vi "pH电极校准.vi"() -> ()   [LabVIEW 2016, in "斯坦道多参数.lvlib"]
uses:
  <vilib>/Utility/miscctls.llb/LVPointTypeDef.ctl
  <vilib>/Analysis/NI_AALBase.lvlib
panel:
  out "滤波设定":dbl
  in  "刷新按钮":bool
  out "第三点信号值":dbl
  out "第二点信号值":dbl
  out "第一点信号值":dbl
  out "温度":dbl format="%#.2f"
  out "通讯状态":string
  out "电极状态标志":u16(ring) items=["OK", "第一点校正通过", "第二点校正通过", "校正失败,电极零点超出范围", "校正失败,电极斜率超出范围", "第三点校正通过"]
  in  "三点标液3":u16(ring)=6 caption="标液3" items=["TECH4.00", "TECH7.00", "TECH10.00", "NIST1.68", "NIST4.01", "NIST6.86", "NIST9.18", "NIST12.68"]
  in  "三点标液2":u16(ring)=5 caption="标液2" items=["TECH4.00", "TECH7.00", "TECH10.00", "NIST1.68", "NIST4.01", "NIST6.86", "NIST9.18", "NIST12.68"]
  in  "三点标液1":u16(ring)=4 caption="标液1" items=["TECH4.00", "TECH7.00", "TECH10.00", "NIST1.68", "NIST4.01", "NIST6.86", "NIST9.18", "NIST12.68"]
  out "第三点校准值":dbl
  in  "校准停止":bool
  in  "校准启动":bool
  out "第二点校准值":dbl
  out "第一点校准值":dbl
  out "提示":string
  in  "校准模式":u16(ring) items=["两点校准", "单点校准", "三点校准"]
  out "最小值":sgl format="%#.2f"
  out "最大值":sgl format="%#.2f"
  out "变异系数":dbl format="%#.6f"
  out "standard deviation":dbl caption="标准差" format="%#.2f"
  out "mean":dbl caption="均值" format="%#.2f"
  out "波形图表":sgl(graph) caption="历史曲线"
  out "当前检测值":dbl caption="测量值" format="%#.2f"
  out "标液2":dbl
  out "标液1":dbl
  out "当前信号值":dbl caption="信号值" format="%#.2f"
  out "偏移值补偿":dbl caption="pH偏移修正值" format="%#.2f"
  out "电极斜率":dbl format="%#.6f"
  out "电极零点":dbl format="%#.6f"
  # "酸碱度电极设定"
  # "℃"
  # "mV"
  # "mV"
  # "%"
  # "请选择校准模式:"
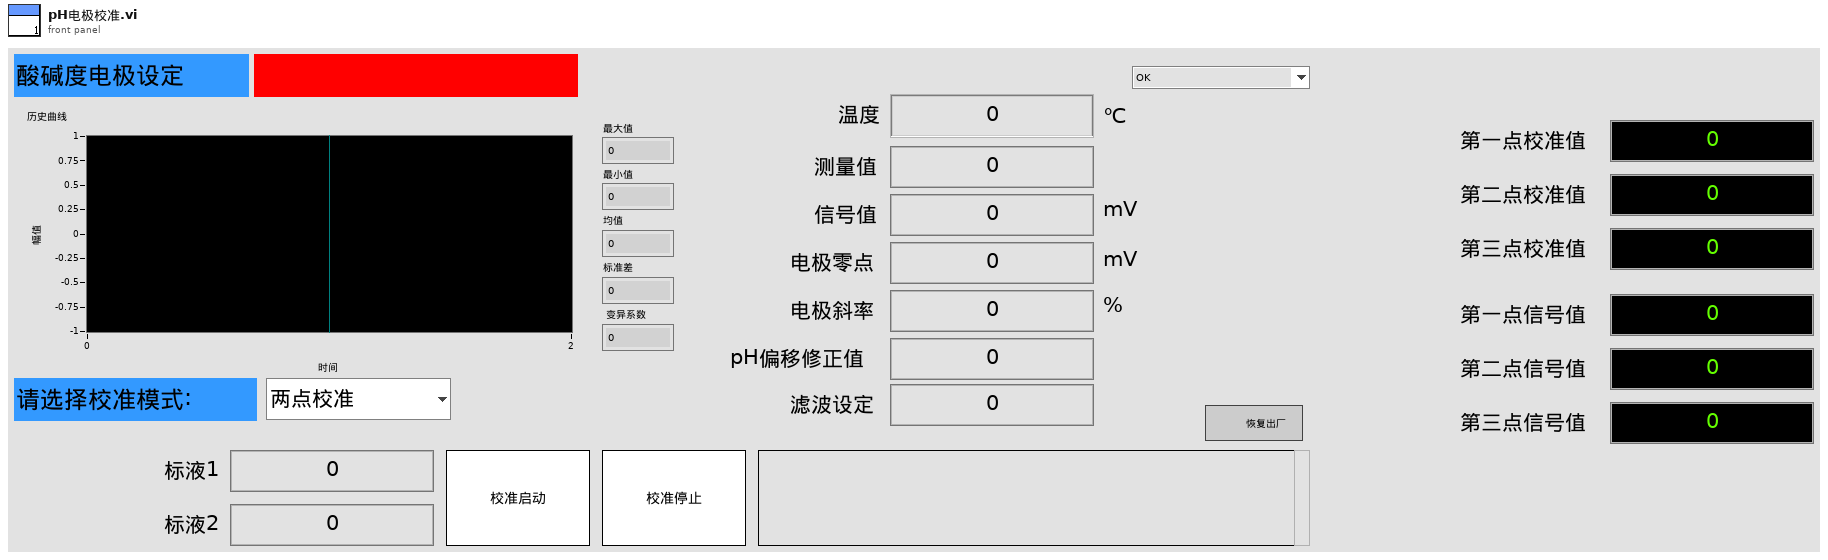
[diagram p1: front panel]
types:
  T1 = typedef "斯坦道多参数.lvlib/通知队列类型.ctl" = enum16{"pH", "DO", "DO2", "Cond", "Turb", "ORP", "叶绿素a", "藻密度", "COD"}
  T2 = typedef "LVPointTypeDef.ctl" = cluster{"Horizontal":i16, "Vertical":i16}
  T3 = cluster{"电极状态标志":u16, "电极型号标志":u16, "酸碱度测量值":sgl, "温度测量值":sgl, "酸碱度信号值":sgl, "温度信号值":sgl, "酸碱度偏移修正值":sgl, "温度偏移修正值":sgl, "手动温度补偿值":sgl, "酸碱度电极零点":sgl, "酸碱度电极斜率":sgl, "第1点标准值记录":sgl, "第1点信号值记录":sgl, "第1点温度值记录":sgl, "第2点标准值记录":sgl, "第2点信号值记录":sgl, "第2点温度值记录":sgl, "命令滤波设定":u16, "温度模式":enum16{"ATC", "MTC"}, "生产批次":u16, "电极序号":u16, "串口地址":u16, "串口波特率":enum16{"9600", "19200", "115200"}, "串口校验位":enum16{"NONE", "ODD", "EVEN"}, "串口停止位":enum16{"1bit", "2bit"}, "第一点标准值":sgl, "第二点标准值":sgl}
  T4 = enum8{"Enabled", "Disabled", "Disabled and Grayed Out"}
  T5 = cluster{"ph":bool, "DO":bool, "Cond":bool, "Turb":bool, "叶绿素a":bool, "藻密度":bool, "ORP":bool, "COD":bool, "DO2":bool}
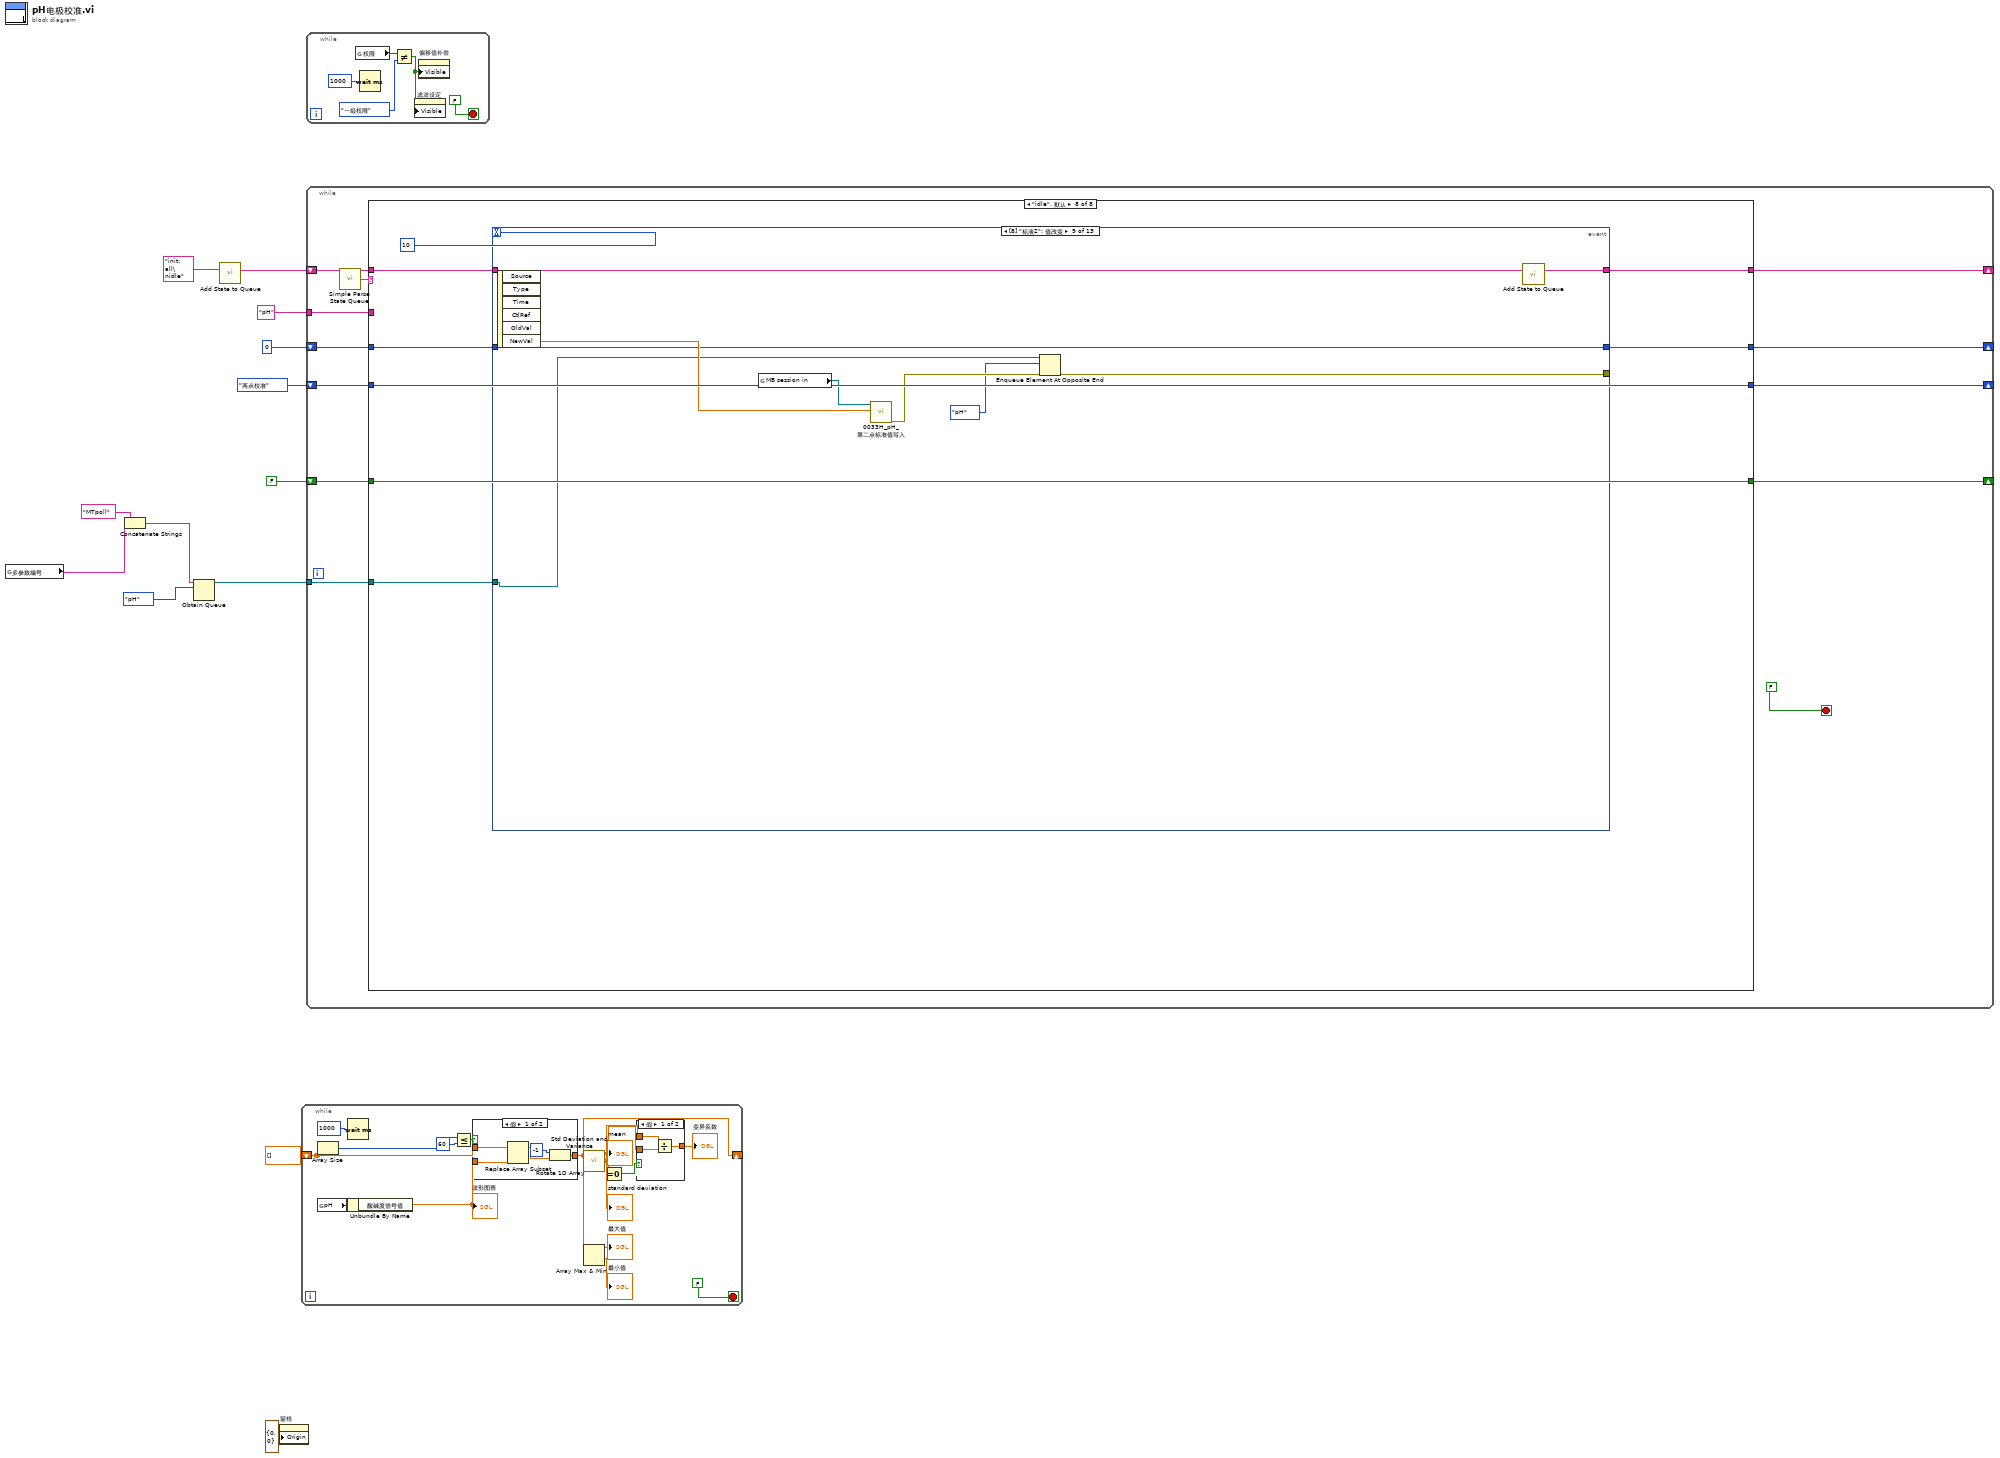
[diagram p0: block diagram]
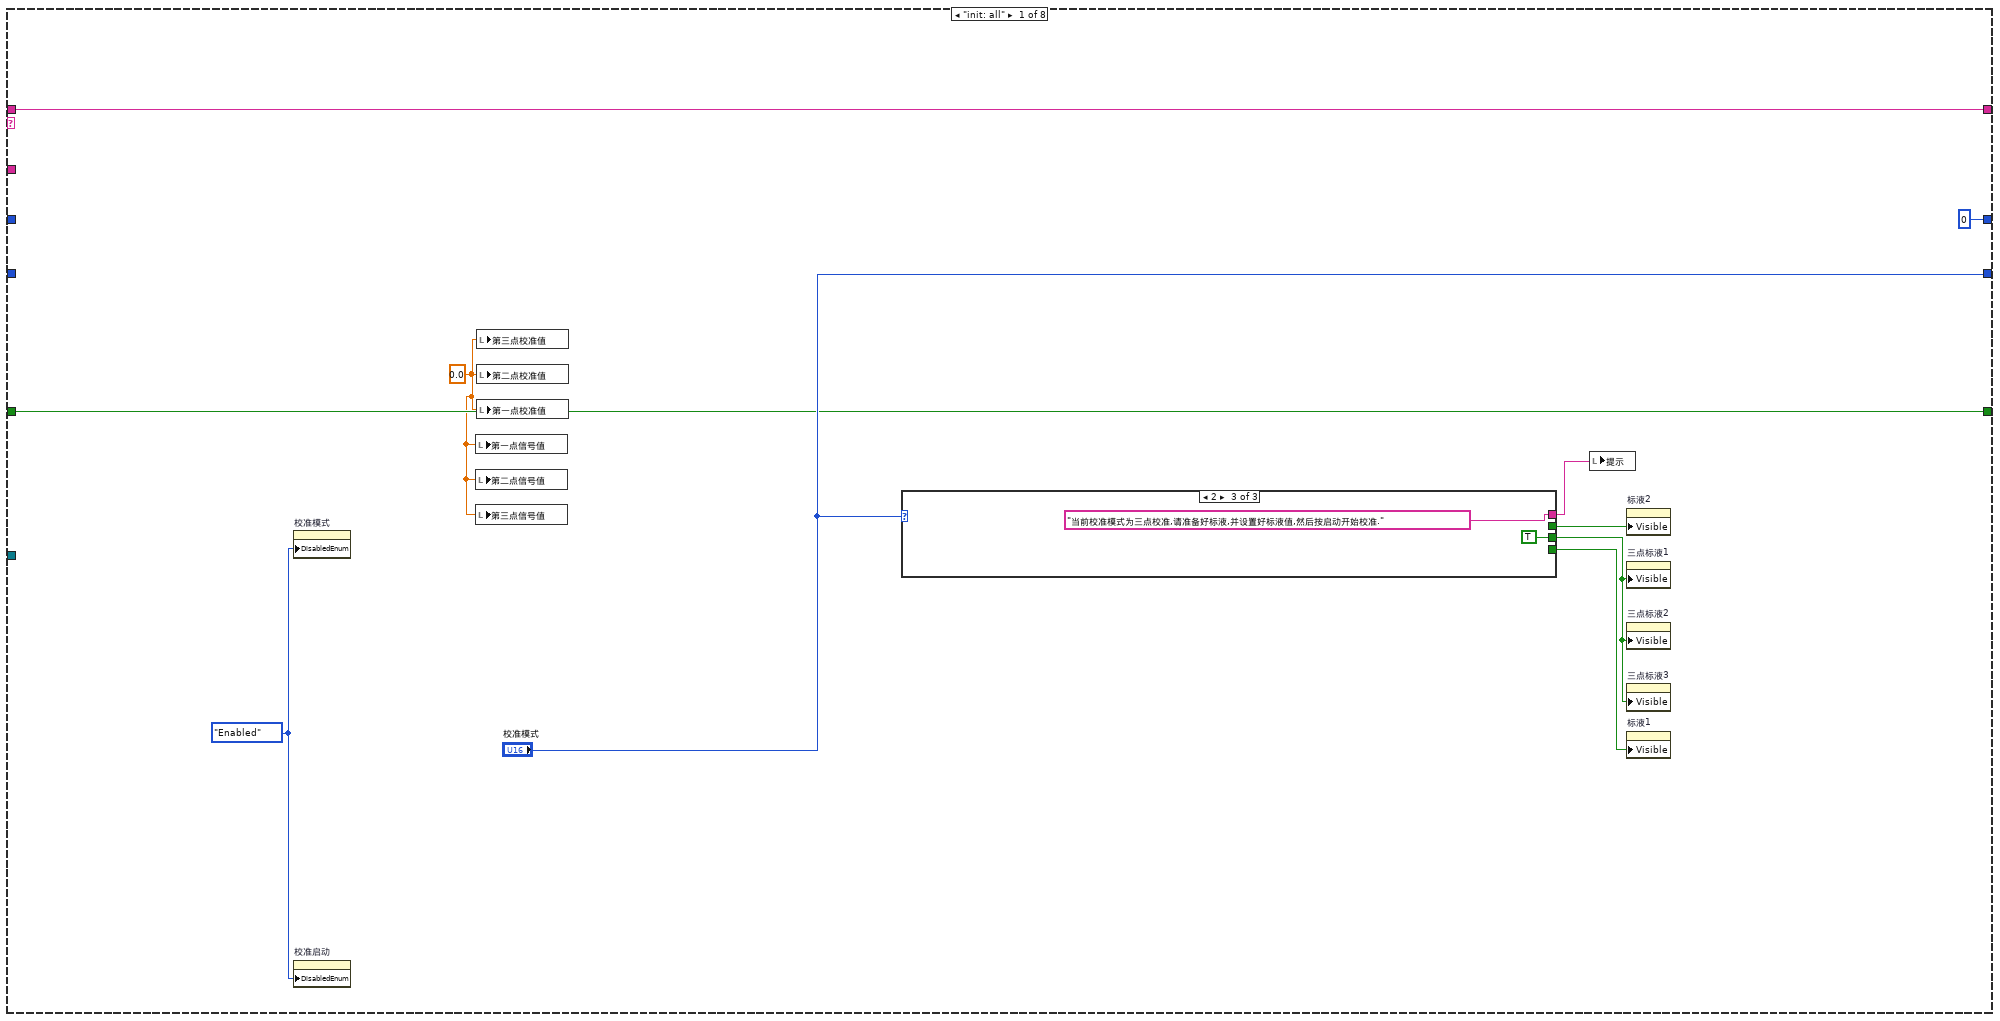
[diagram p2: hidden frame]
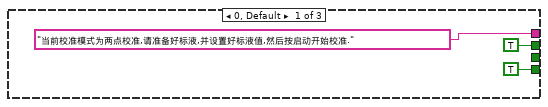
[diagram p3: hidden frame]
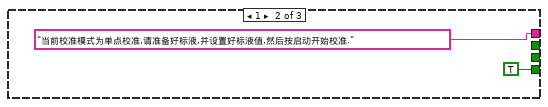
[diagram p4: hidden frame]
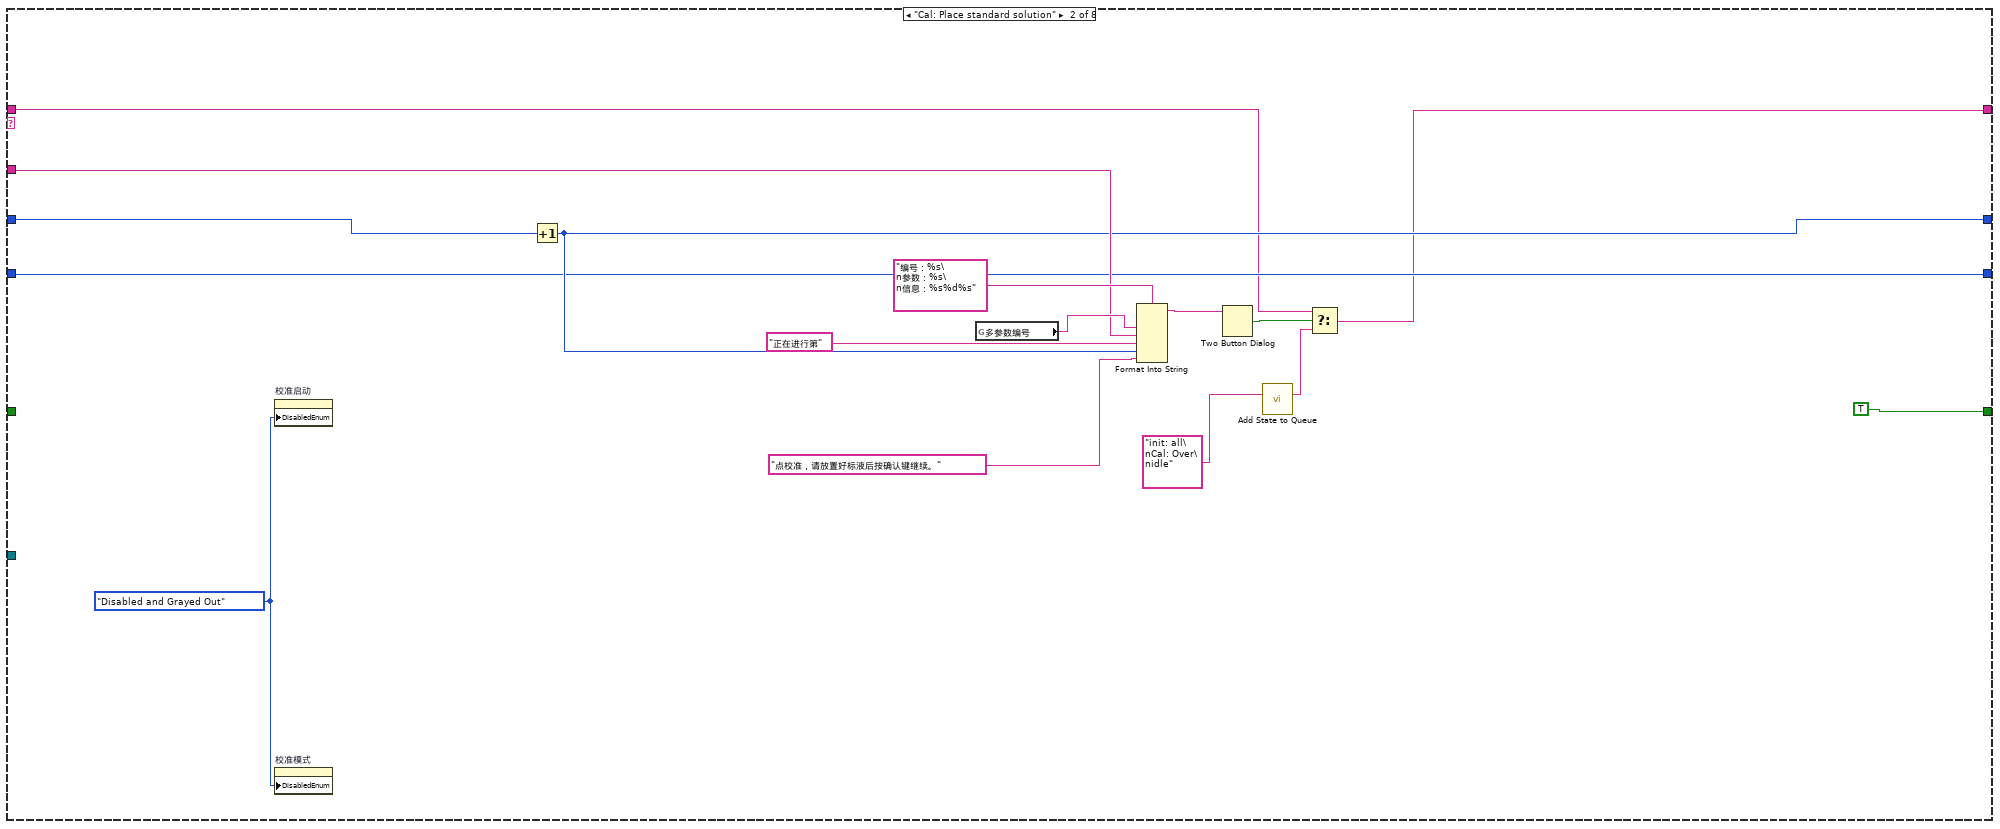
[diagram p5: hidden frame]
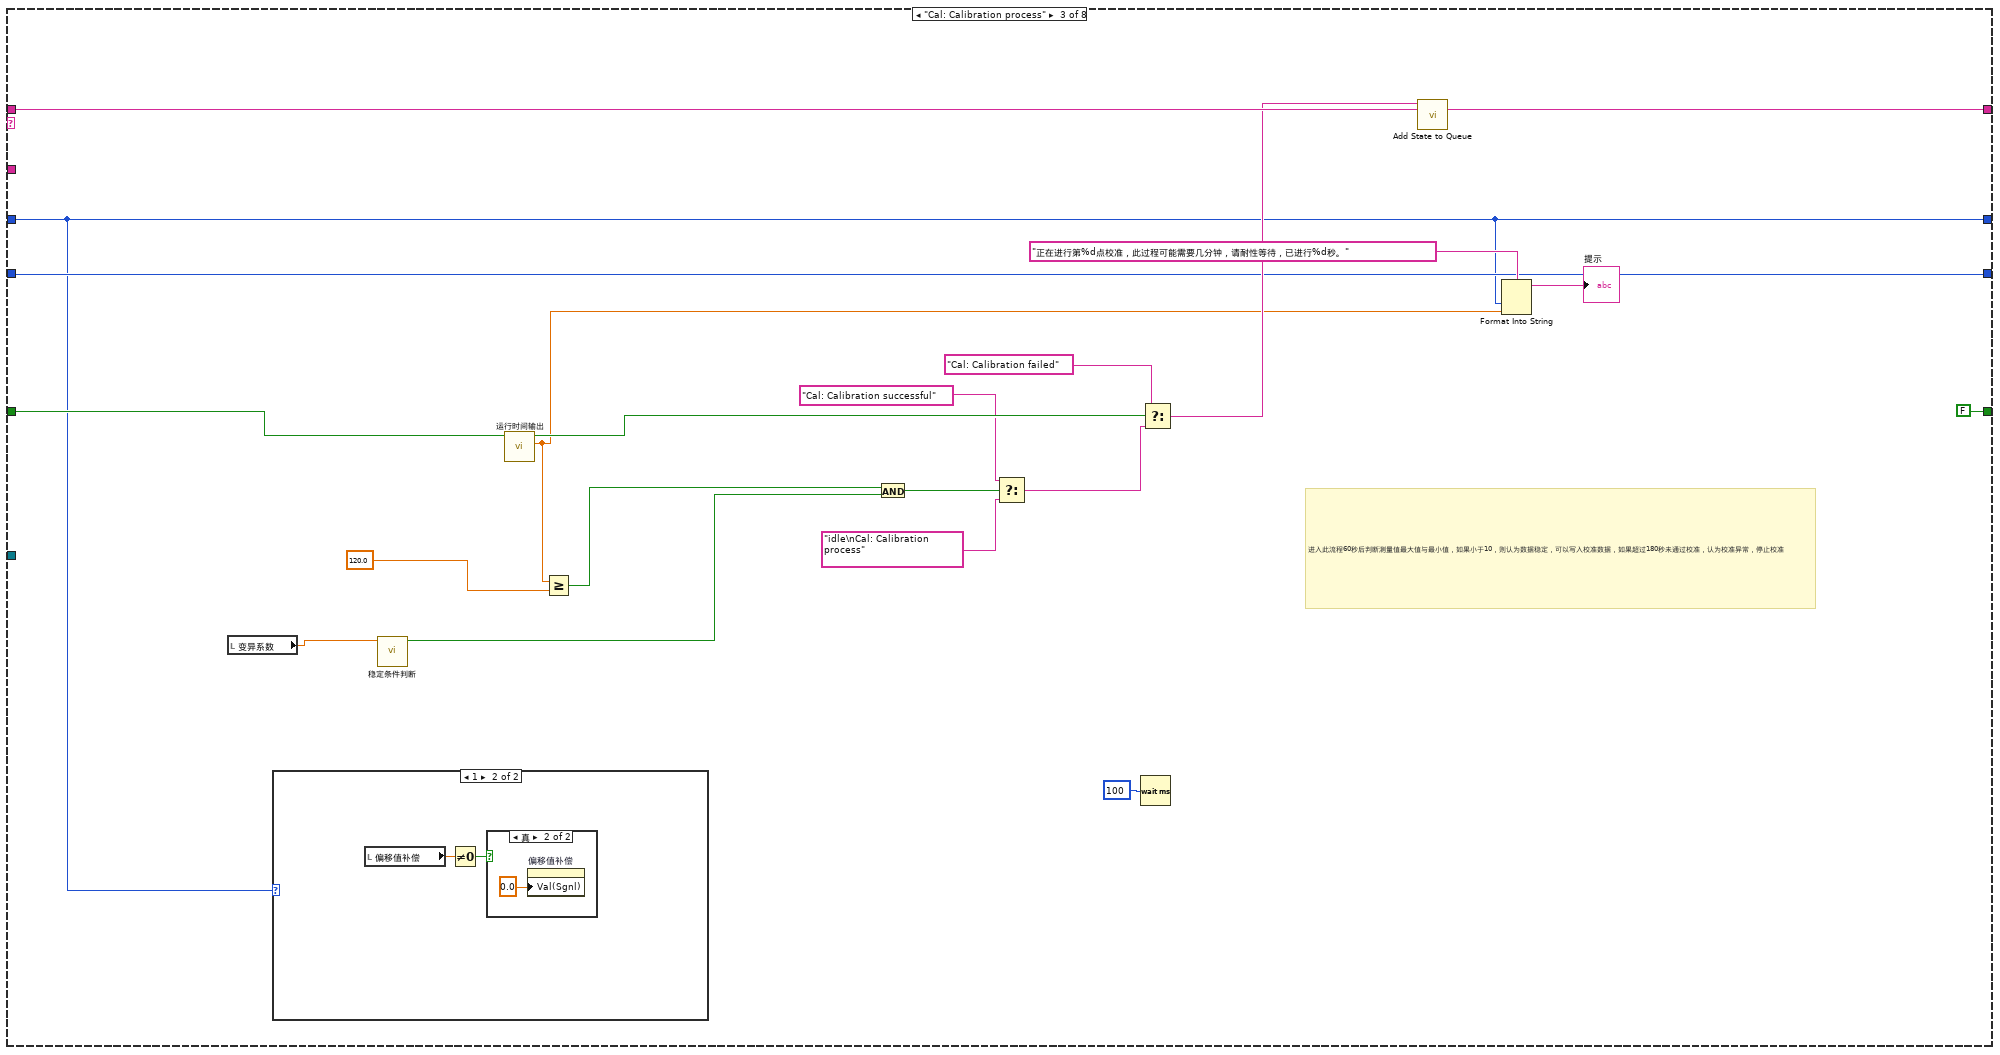
[diagram p6: hidden frame]
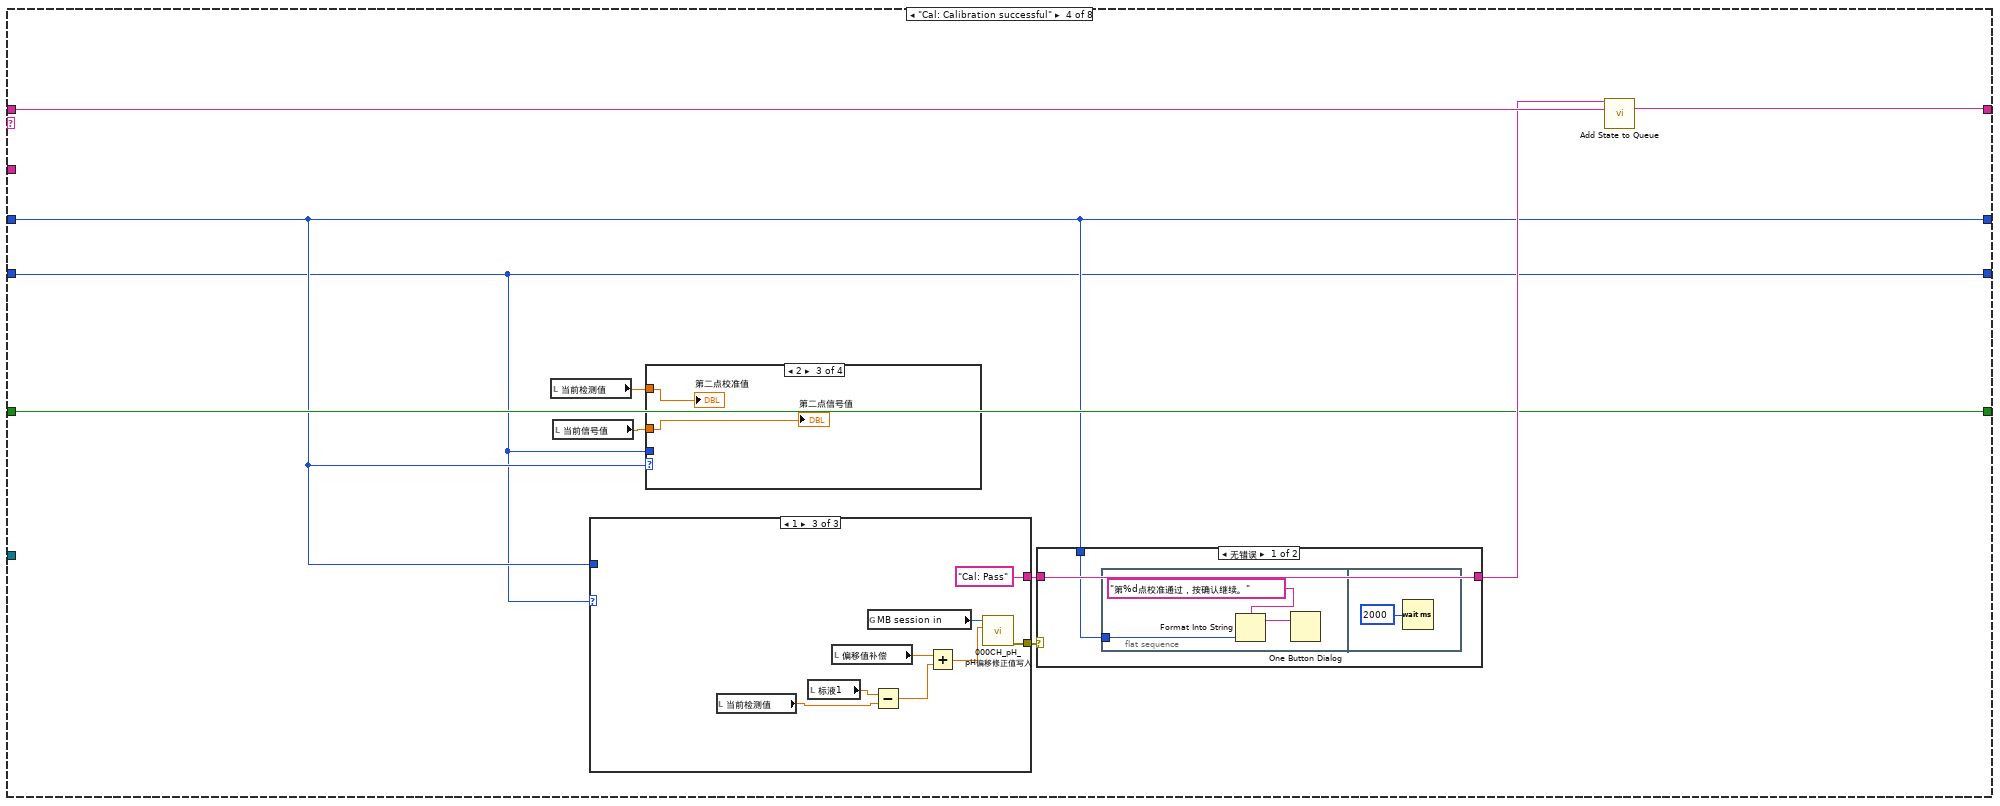
[diagram p9: hidden frame]
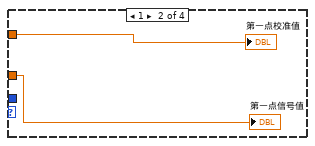
[diagram p11: hidden frame]
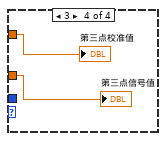
[diagram p12: hidden frame]
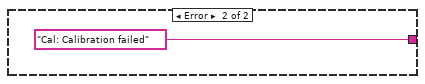
[diagram p13: hidden frame]
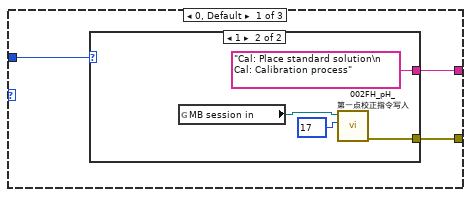
[diagram p14: hidden frame]
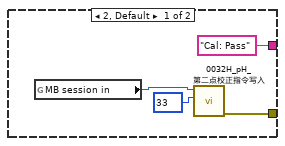
[diagram p15: hidden frame]
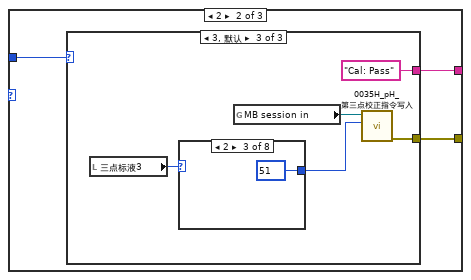
[diagram p16: hidden frame]
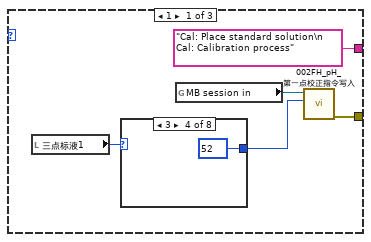
[diagram p17: hidden frame]
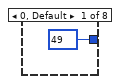
[diagram p18: hidden frame]
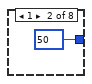
[diagram p19: hidden frame]
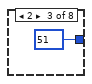
[diagram p20: hidden frame]
diagram:
  n1 = global read "多参数全局变量.vi" "多参数编号"() -> (w3:string)
  n2 = Concatenate Strings("MTpoll" ("名称（未命名）"), w3) -> (w4:string)
  n3 = Obtain Queue(name (unnamed)=w4, element data type=通知队列类型."pH" ("枚举")) -> (queue out=w2:refnum<queue>)  [unwired: 3 in, 2 out]
  n4 = call "Add State to Queue.vi"("State(s) In (\"\")"="init: all\nidle" ("State(s) In (\"\")")) -> ("States Out"=w10:string)  [unwired: 14 in]
  n5 = property on="窗格" class="Pane"("Origin"=T2 {"Horizontal"=0, "Vertical"=0} ("原点")) -> ()  [unwired: 2 in, 2 out]
  n6 = while {
    shift-right: [w20] -> _
    shift-left: sgl[] [] -> [w24]
    stop <- FALSE stop-if-true
    n7 = Array Size(array=w24) -> (size(s)=w26:i32)
    n8 = global read "国弘过程全局变量.vi" "pH"() -> (w21:T3)
    n9 = Wait (ms)(milliseconds to wait=u32 1000 ("等待时间（毫秒）")) -> ()  [unwired: 1 out]
    n10 = Unbundle By Name(w21) -> ("酸碱度信号值"=w14:sgl)
    "波形图表" <- w14
    n11 = Less Or Equal?(x=w26, y=60) -> (x <= y?=w25:bool)
    n12 = case shown="假" w25 {
      tunnel: w24 -> [w36 w39]
      tunnel: w14 -> [w34 w38]
      tunnel: [w32 w37] -> w20
      frame False {
        n13 = Replace Array Subset(array=w36, new element=w34) -> (w35:sgl[])  [unwired: 1 in]
        n14 = Rotate 1D Array(1:w35, 2:-1 ("n")) -> (0:w32:sgl[])
      }
      frame True {
        n15 = Insert Into Array(array=w39, new element=w38) -> (w37:sgl[])  [unwired: 1 in]
      }
    }
    n16 = call <vilib>:"Std Deviation and Variance.vi"("X"=w20) -> ("mean"=w16:dbl, "standard deviation"=w15:dbl)  [unwired: 1 in, 1 out]
    "mean" <- w16
    "standard deviation" <- w15
    n17 = Array Max & Min(array=w20) -> (max value=→"最大值":sgl, min value=→"最小值":sgl)  [unwired: 2 out]
    n18 = Equal To 0?(x=w16) -> (x = 0?=w23:bool)
    n19 = case shown="假" w23 {
      tunnel: w15 -> [w31 _]
      tunnel: [w30 _] -> w17
      tunnel: w16 -> [w29 _]
      frame False {
        n20 = Divide(x=w31, y=w29) -> (x/y=w30:dbl)
      }
      frame True {
      }
    }
    "变异系数" <- w17
  }
  n21 = while {
    shift-right: [w48] -> _
    shift-left: w10 -> [w52]
    shift-right: [w45] -> _
    shift-left: 0 -> [w47]
    tunnel: "pH" ("State(s) In (\"\")") -> [w46]
    shift-right: [w43] -> _
    shift-left: enum16{"两点校准", "单点校准", "三点校准"}."两点校准" ("校准模式") -> [w44]
    shift-right: [w41] -> _
    shift-left: FALSE -> [w42]
    tunnel: w2 -> [w40]
    stop <- FALSE stop-if-true
    n22 = call "Simple Parse State Queue.vi"("State Queue"=w52) -> ("Remain States"=w49:string, "Next State"=w50:string)  [unwired: 13 in]
    n23 = case shown="\"idle\", 默认" w50 {
      tunnel: w49 -> [w62 w72 w105 w117 _ _ w262 w273]
      tunnel: [w62 w71 w104 w116 w201 w208 w262 w272] -> w48
      tunnel: w47 -> [_ w81 w89 w111 w204 w217 w261 w270]
      tunnel: w46 -> [_ w82 _ _ w195 w213 _ _]
      tunnel: [0 w79 w89 w111 w204 w217 w261 w271] -> w45
      tunnel: w44 -> [_ w78 w90 w110 w203 w209 w260 w269]
      tunnel: ["校准模式" w78 w90 w110 w203 w209 w260 w269] -> w43
      tunnel: w42 -> [w55 _ w92 w112 w202 w212 w259 w267]
      tunnel: [w55 TRUE FALSE w112 w202 w212 w259 w267] -> w41
      tunnel: w40 -> [_ _ _ _ _ _ _ w266]
      frame "init: all" {
        w54 = T4."Enabled" ("禁用")
        w53 = 0.0 ("第一点校准值")
        n24 = property on="校准模式" class="Ring (严格)"("DisabledEnum"=w54) -> ()  [unwired: 2 in, 2 out]
        n25 = property on="校准启动" class="Bool"("DisabledEnum"=w54) -> ()  [unwired: 2 in, 2 out]
        n26 = local write "第一点信号值"(w53) -> ()
        n27 = local write "第二点信号值"(w53) -> ()
        n28 = local write "第三点信号值"(w53) -> ()
        n29 = local write "第三点校准值"(w53) -> ()
        n30 = local write "第二点校准值"(w53) -> ()
        n31 = local write "第一点校准值"(w53) -> ()
        n32 = case shown="2" "校准模式" {
          tunnel: ["当前校准模式为两点校准,请准备好标液,并设置好标液值,然后按启动开始校准." ("提示") "当前校准模式为单点校准,请准备好标液,并设置好标液值,然后按启动开始校准." ("提示") "当前校准模式为三点校准,请准备好标液,并设置好标液值,然后按启动开始校准." ("提示")] -> w57
          tunnel: [TRUE ("可见") _ _] -> w61
          tunnel: [TRUE ("可见") TRUE ("可见") _] -> w59
          tunnel: [_ _ TRUE ("可见")] -> w60
          frame 0, Default {
          }
          frame 1 {
          }
          frame 2 {
          }
        }
        n33 = local write "提示"(w57) -> ()
        n34 = property on="标液2" class="DigNum (严格)"("Visible"=w61) -> ()  [unwired: 2 in, 2 out]
        n35 = property on="三点标液1" class="Ring (严格)"("Visible"=w60) -> ()  [unwired: 2 in, 2 out]
        n36 = property on="三点标液2" class="Ring (严格)"("Visible"=w60) -> ()  [unwired: 2 in, 2 out]
        n37 = property on="三点标液3" class="Ring (严格)"("Visible"=w60) -> ()  [unwired: 2 in, 2 out]
        n38 = property on="标液1" class="DigNum (严格)"("Visible"=w59) -> ()  [unwired: 2 in, 2 out]
      }
      frame "Cal: Place standard solution" {
        w76 = T4."Disabled and Grayed Out" ("禁用")
        n39 = property on="校准启动" class="Bool"("DisabledEnum"=w76) -> ()  [unwired: 2 in, 2 out]
        n40 = property on="校准模式" class="Ring (严格)"("DisabledEnum"=w76) -> ()  [unwired: 2 in, 2 out]
        n41 = Increment(x=w81) -> (x+1=w79:i32)
        n42 = global read "多参数全局变量.vi" "多参数编号"() -> (w84:string)
        n43 = Format Into String(format string="编号：%s\n参数：%s\n信息：%s%d%s" ("格式字符串"), w84, w82, "正在进行第" ("消息"), w79, "点校准，请放置好标液后按确认键继续。" ("消息")) -> (resulting string=w75:string)  [unwired: 2 in, 1 out]
        n44 = Two Button Dialog(message=w75) -> (T button?=w74:bool)  [unwired: 2 in]
        n45 = call "Add State to Queue.vi"("State(s) In (\"\")"="init: all\nCal: Over\nidle" ("State(s) In (\"\")")) -> ("States Out"=w73:string)  [unwired: 14 in]
        n46 = Select(t=w72, s=w74, f=w73) -> (s? t:f=w71:string)
      }
      frame "Cal: Calibration process" {
        # "进入此流程60秒后判断测量值最大值与最小值，如果小于10，则认为数据稳定，可以写入校准数据，如果超过180秒未通过校准，认为校准异常，停止校准"
        n47 = local read "变异系数"() -> (w87:dbl)
        n48 = case shown="1" w89 {
          frame 0, Default {
          }
          frame 1 {
            n49 = local read "偏移值补偿"() -> (w107:dbl)
            n50 = Not Equal To 0?(x=w107) -> (x != 0?=w108:bool)
            n51 = case shown="真" w108 {
              frame False {
              }
              frame True {
                n52 = property on="偏移值补偿" class="DigNum (严格)"("Val(Sgnl)"=0.0 ("值(信号)")) -> ()  [unwired: 2 in, 2 out]
              }
            }
          }
        }
        n53 = call "稳定条件判断.vi"("变异系数"=w87) -> ("布尔"=w86:bool)  [unwired: 10 in]
        n54 = call "运行时间输出.vi"("初始化"=w92) -> ("Elapsed Time (s)"=w88:dbl, "Time has Elapsed"=w106:bool)  [unwired: 9 in]
        n55 = Greater Or Equal?(x=w88, y=120.0) -> (x >= y?=w101:bool)
        n56 = And(x=w101, y=w86) -> (x .and. y?=w98:bool)
        n57 = Select(t="Cal: Calibration successful" ("State(s) In (\"\")"), s=w98, f="idle\nCal: Calibration process" ("State(s) In (\"\")")) -> (s? t:f=w97:string)
        n58 = Wait (ms)(milliseconds to wait=u32 100 ("等待时间（毫秒）")) -> ()  [unwired: 1 out]
        n59 = Select(t="Cal: Calibration failed" ("State(s) In (\"\")"), s=w106, f=w97) -> (s? t:f=w96:string)
        n60 = call "Add State to Queue.vi"("State(s) In Front (\"\")"=w96, "State(s) In (\"\")"=w105) -> ("States Out"=w104:string)  [unwired: 13 in]
        n61 = Format Into String(format string="正在进行第%d点校准，此过程可能需要几分钟，请耐性等待，已进行%d秒。" ("格式字符串"), w89, w88) -> (resulting string=→"提示":string)  [unwired: 2 in, 1 out]
      }
      frame "Cal: Calibration successful" {
        n62 = local read "当前检测值"() -> (w113:dbl)
        n63 = local read "当前信号值"() -> (w114:dbl)
        n64 = case shown="1" w110 {
          tunnel: [w135 w146 w188] -> w119
          tunnel: [w134 w144 "Cal: Pass" ("State(s) In (\"\")")] -> w118
          tunnel: w111 -> [w133 w145 _]
          frame 0, Default {
            n65 = case shown="1" w133 {
              tunnel: [w136 w141] -> w135
              tunnel: ["Cal: Pass" ("State(s) In (\"\")") "Cal: Place standard solution\n Cal: Calibration process" ("State(s) In (\"\")")] -> w134
              frame 2, Default {
                n66 = global read "多参数全局变量.vi" "MB session in"() -> (w138:refnum<class "MB_Master.lvclass">)
                n67 = call "0032H_pH_第二点校正指令写入.vi"("数值"=u16 33, "MB session in"=w138) -> ("error out"=w136:errorcluster)  [unwired: 8 in, 1 out]
              }
              frame 1 {
                n68 = global read "多参数全局变量.vi" "MB session in"() -> (w143:refnum<class "MB_Master.lvclass">)
                n69 = call "002FH_pH_第一点校正指令写入.vi"("数值"=u16 17, "MB session in"=w143) -> ("error out"=w141:errorcluster)  [unwired: 8 in, 1 out]
              }
            }
          }
          frame 2 {
            n70 = case shown="3, 默认" w145 {
              tunnel: [w148 w161 w174] -> w146
              tunnel: ["Cal: Place standard solution\n Cal: Calibration process" ("State(s) In (\"\")") "Cal: Place standard solution\n Cal: Calibration process" ("State(s) In (\"\")") "Cal: Pass" ("State(s) In (\"\")")] -> w144
              frame 1 {
                n71 = local read "三点标液1"() -> (w150:u16)
                n72 = case shown="3" w150 {
                  tunnel: [u16 49 ("数值") u16 50 ("数值") u16 51 ("数值") u16 52 ("数值") u16 53 ("数值") u16 54 ("数值") u16 55 ("数值") u16 56 ("数值")] -> w149
                  frame 0, Default {
                  }
                  frame 1 {
                  }
                  frame 2 {
                  }
                  frame 3 {
                  }
                  frame 4 {
                  }
                  frame 5 {
                  }
                  frame 6 {
                  }
                  frame 7 {
                  }
                }
                n73 = global read "多参数全局变量.vi" "MB session in"() -> (w151:refnum<class "MB_Master.lvclass">)
                n74 = call "002FH_pH_第一点校正指令写入.vi"("数值"=w149, "MB session in"=w151) -> ("error out"=w148:errorcluster)  [unwired: 8 in, 1 out]
              }
              frame 2 {
                n75 = local read "三点标液2"() -> (w163:u16)
                n76 = case shown="7" w163 {
                  tunnel: [u16 49 ("数值") u16 50 ("数值") u16 51 ("数值") u16 52 ("数值") u16 53 ("数值") u16 54 ("数值") u16 55 ("数值") u16 56 ("数值")] -> w162
                  frame 0, Default {
                  }
                  frame 1 {
                  }
                  frame 2 {
                  }
                  frame 3 {
                  }
                  frame 4 {
                  }
                  frame 5 {
                  }
                  frame 6 {
                  }
                  frame 7 {
                  }
                }
                n77 = global read "多参数全局变量.vi" "MB session in"() -> (w164:refnum<class "MB_Master.lvclass">)
                n78 = call "0032H_pH_第二点校正指令写入.vi"("数值"=w162, "MB session in"=w164) -> ("error out"=w161:errorcluster)  [unwired: 8 in, 1 out]
              }
              frame 3, Default {
                n79 = local read "三点标液3"() -> (w176:u16)
                n80 = case shown="2" w176 {
                  tunnel: [u16 49 ("数值") u16 50 ("数值") u16 51 ("数值") u16 52 ("数值") u16 53 ("数值") u16 54 ("数值") u16 55 ("数值") u16 56 ("数值")] -> w175
                  frame 0, Default {
                  }
                  frame 1 {
                  }
                  frame 2 {
                  }
                  frame 3 {
                  }
                  frame 4 {
                  }
                  frame 5 {
                  }
                  frame 6 {
                  }
                  frame 7 {
                  }
                }
                n81 = global read "多参数全局变量.vi" "MB session in"() -> (w177:refnum<class "MB_Master.lvclass">)
                n82 = call "0035H_pH_第三点校正指令写入.vi"("数值"=w175, "MB session in"=w177) -> ("error out"=w174:errorcluster)  [unwired: 8 in, 1 out]
              }
            }
          }
          frame 1 {
            n83 = local read "当前检测值"() -> (w186:dbl)
            n84 = local read "标液1"() -> (w193:dbl)
            n85 = local read "偏移值补偿"() -> (w189:dbl)
            n86 = global read "多参数全局变量.vi" "MB session in"() -> (w192:refnum<class "MB_Master.lvclass">)
            n87 = Subtract(x=w193, y=w186) -> (x-y=w191:dbl)
            n88 = Add(x=w189, y=w191) -> (x+y=w190:dbl)
            n89 = call "000CH_pH_pH偏移修正值写入.vi"("数值"=w190, "MB session in"=w192) -> ("error out"=w188:errorcluster)  [unwired: 8 in, 1 out]
          }
        }
        n90 = case shown="2" w111 {
          tunnel: w114 -> [_ w121 w122 w124]
          tunnel: w113 -> [_ w120 w123 w125]
          tunnel: w110 -> [_ _ _ _]
          frame 0, Default {
          }
          frame 1 {
            "第一点校准值" <- w120
            "第一点信号值" <- w121
          }
          frame 2 {
            "第二点校准值" <- w123
            "第二点信号值" <- w122
          }
          frame 3 {
            "第三点校准值" <- w125
            "第三点信号值" <- w124
          }
        }
        n91 = case shown="无错误" w119 {
          tunnel: w118 -> [w127 _]
          tunnel: [w127 "Cal: Calibration failed" ("State(s) In (\"\")")] -> w115
          tunnel: w111 -> [w126 _]
          frame No Error {
            n92 = flat-sequence {
              tunnel: w126 -> [w128]
              frame #0 {
                n93 = Format Into String(format string="第%d点校准通过，按确认继续。" ("格式字符串"), w128) -> (resulting string=w130:string)  [unwired: 2 in, 1 out]
                n94 = One Button Dialog(message=w130) -> ()  [unwired: 1 in, 1 out]
              }
              frame #1 {
                n95 = Wait (ms)(milliseconds to wait=u32 2000 ("等待时间（毫秒）")) -> ()  [unwired: 1 out]
              }
            }
          }
          frame Error {
          }
        }
        n96 = call "Add State to Queue.vi"("State(s) In Front (\"\")"=w115, "State(s) In (\"\")"=w117) -> ("States Out"=w116:string)  [unwired: 13 in]
      }
      frame "Cal: Calibration failed" {
        n97 = global read "多参数全局变量.vi" "多参数编号"() -> (w198:string)
        n98 = call "Add State to Queue.vi"("State(s) In (\"\")"="init: all\nCal: Over\nidle" ("State(s) In (\"\")")) -> ("States Out"=w201:string)  [unwired: 14 in]
        n99 = Format Into String(format string="编号：%s\n参数：%s\n信息：%s" ("格式字符串"), w198, w195, "校准失败！" ("消息")) -> (resulting string=w197:string)  [unwired: 2 in, 1 out]
        n100 = One Button Dialog(message=w197) -> ()  [unwired: 1 in, 1 out]
        n101 = call "校准日志.vi"("table"="校准记录", "日志信息"=w197) -> ()  [unwired: 9 in, 1 out]
      }
      frame "Cal: Pass" {
        n102 = flat-sequence {
          tunnel: [w222] -> w210
          tunnel: w209 -> [w221]
          tunnel: [w220] -> w207
          tunnel: [w219] -> w206
          frame #0 {
            n103 = Wait (ms)(milliseconds to wait=u32 3000 ("等待时间（毫秒）")) -> ()  [unwired: 1 out]
          }
          frame #1 {
            n104 = global read "国弘过程全局变量.vi" "pH"() -> (w223:T3)
            n105 = Unbundle By Name(w223) -> ("电极状态标志"=w224:u16, "酸碱度电极零点"=w220:sgl, "酸碱度电极斜率"=w219:sgl)
            n106 = case shown="0, 默认" w221 {
              tunnel: [w226 w241 w258] -> w222
              tunnel: w224 -> [w225 w240 _]
              frame 0, Default {
                n107 = case shown="2" w225 {
                  selector: w225 -> [_ _ w237]
                  tunnel: ["校准异常，校准未完成。" ("格式字符串") w235 w236] -> w226
                  frame 0, Default {
                  }
                  frame 2 {
                    n108 = local read "第一点校准值"() -> (w233:dbl)
                    n109 = local read "第一点信号值"() -> (w234:dbl)
                    n110 = local read "第二点校准值"() -> (w230:dbl)
                    n111 = local read "第二点信号值"() -> (w229:dbl)
                    n112 = local read "标液1"() -> (w231:dbl)
                    n113 = local read "标液2"() -> (w228:dbl)
                    n114 = Format Into String(format string="校准结果：\n第一点校准值=%#.2f，第一点信号值=%#.2f mV，第一点标准值=%#.2f；\n第二点校准值=%#.2f，第二点信号值=%#.2f mV，第二点标准值=%#.2f。" ("提示"), w233, w234, w231, w230, w229, w228) -> (resulting string=w235:string)  [unwired: 2 in, 1 out]
                  }
                  frame 3, 4 {
                    n115 = case shown="4" w237 {
                      tunnel: ["校正失败，电极零点超出范围" "校正失败，电极斜率超出范围"] -> w236
                      frame 3, Default {
                      }
                      frame 4 {
                      }
                    }
                  }
                }
              }
              frame 2 {
                n116 = case shown="5" w240 {
                  tunnel: ["校准异常，校准未完成。" ("格式字符串") w253] -> w241
                  frame 0, Default {
                  }
                  frame 5 {
                    n117 = local read "第一点校准值"() -> (w252:dbl)
                    n118 = local read "第一点信号值"() -> (w250:dbl)
                    n119 = local read "第二点校准值"() -> (w248:dbl)
                    n120 = local read "第二点信号值"() -> (w247:dbl)
                    n121 = local read "第三点校准值"() -> (w245:dbl)
                    n122 = local read "第三点信号值"() -> (w244:dbl)
                    n123 = property on="三点标液1" class="Ring (严格)"() -> ("RingText.Text"=w249:string)  [unwired: 2 in, 2 out]
                    n124 = property on="三点标液2" class="Ring (严格)"() -> ("RingText.Text"=w246:string)  [unwired: 2 in, 2 out]
                    n125 = property on="三点标液3" class="Ring (严格)"() -> ("RingText.Text"=w243:string)  [unwired: 2 in, 2 out]
                    n126 = Format Into String(format string="校准结果：\n第一点校准值=%#.2f，第一点信号值=%#.2f mV，第一点标准值=%s；\n第二点校准值=%#.2f，第二点信号值=%#.2f mV，第二点标准值=%s；\n第三点校准值=%#.2f，第三点信号值=%#.2f mV，第三点标准值=%s。" ("提示"), w252, w250, w249, w248, w247, w246, w245, w244, w243) -> (resulting string=w253:string)  [unwired: 2 in, 1 out]
                  }
                }
              }
              frame 1 {
                n127 = local read "第一点校准值"() -> (w257:dbl)
                n128 = local read "第一点信号值"() -> (w255:dbl)
                n129 = local read "标液1"() -> (w254:dbl)
                n130 = Format Into String(format string="校准结果：\n校准值=%#.2f，信号值=%#.2f，标准值=%#.2f。" ("提示"), w257, w255, w254) -> (resulting string=w258:string)  [unwired: 2 in, 1 out]
              }
            }
          }
        }
        n131 = call "Add State to Queue.vi"("State(s) In (\"\")"="init: all\nCal: Over\nidle" ("State(s) In (\"\")")) -> ("States Out"=w208:string)  [unwired: 14 in]
        n132 = global read "多参数全局变量.vi" "多参数编号"() -> (w214:string)
        n133 = Format Into String(format string="编号：%s\n参数：%s\n信息：%s\n电极零点=%#.2f，电极斜率=%#.2f%%。" ("格式字符串"), w214, w213, w210, w207, w206) -> (resulting string=w211:string)  [unwired: 2 in, 1 out]
        n134 = One Button Dialog(message=w211) -> ()  [unwired: 1 in, 1 out]
        n135 = call "校准日志.vi"("table"="校准记录", "日志信息"=w211) -> ()  [unwired: 9 in, 1 out]
      }
      frame "Cal: Over" {
        n136 = global read "多参数全局变量.vi" "校准运行状态"() -> (w264:T5)
        n137 = Bundle By Name(cluster=w264, "ph"=FALSE) -> (w265:T5)
        n138 = global write "多参数全局变量.vi" "校准运行状态"(w265) -> ()
      }
      frame "idle", Default {
        n139 = event shown="[8] \"标液2\": 值改变" {
          selector: _ -> [_ _ _ _ _ _ _ _ _ _ _ _ _]
          dyn-events: _ -> [_ _ _ _ _ _ _ _ _ _ _ _ _]
          timeout: 10 -> [_ _ _ _ _ _ _ _ _ _ _ _ _]
          tunnel: [_ _ _ _ _ _ w358 w368 w377 w386 _ _ _] -> _
          tunnel: w273 -> [w291 w295 w296 w318 w332 w353 w365 w369 w378 w390 w395 w406 _]
          tunnel: [w290 w294 w297 w319 w333 w354 w364 w370 w379 w391 w394 w405 w408] -> w272
          tunnel: [w289 w292 w298 w320 w334 w355 w363 w371 w380 w392 w393 w403 w409] -> w271
          tunnel: w270 -> [w289 w292 w298 w320 w334 w355 w363 w371 w380 w392 w393 w403 w409]
          tunnel: w266 -> [_ _ _ _ _ _ w360 w367 w376 w385 _ _ _]
          event Timeout {
            n140 = event-data() -> ()  [unwired: 1 in, 3 out]
            n141 = global read "国弘过程全局变量.vi" "pH"() -> (w288:T3)
            n142 = Unbundle By Name(w288) -> ("电极状态标志"=→"电极状态标志":u16, "酸碱度电极零点"=→"电极零点":sgl, "酸碱度电极斜率"=→"电极斜率":sgl, "酸碱度偏移修正值"=→"偏移值补偿":sgl, "酸碱度信号值"=→"当前信号值":sgl, "第一点标准值"=→"标液1":sgl, "第二点标准值"=→"标液2":sgl, "酸碱度测量值"=→"当前检测值":sgl, "温度测量值"=→"温度":sgl, "命令滤波设定"=→"滤波设定":u16)  [unwired: 1 out]
            n143 = global read "多参数全局变量.vi" "ph通讯状态"() -> (w277:bool)
            n144 = property on="通讯状态" class="Str"("Blinking"=TRUE ("闪烁"), "Text.BG Color"=u32 16711680, "Visible"=w277) -> ()  [unwired: 2 in, 2 out]
            n145 = call "Add State to Queue.vi"("State(s) In (\"\")"=w291) -> ("States Out"=w290:string)  [unwired: 14 in]
            "通讯状态" <- "通讯异常" ("当前串口")
          }
          event "校准模式": Value Change {
            n146 = event-data() -> ()  [unwired: 1 in, 6 out]
            n147 = call "Add State to Queue.vi"("State(s) In (\"\")"=w295, "State(s) At Back (\"\")"="init: all\nidle" ("State(s) In (\"\")")) -> ("States Out"=w294:string)  [unwired: 13 in]
          }
          event "三点标液1": Value Change {
            n148 = event-data() -> ("NewVal"=w299:u16)  [unwired: 1 in, 5 out]
            n149 = case shown="1" w299 {
              frame 0, Default {
                w300 = u16 0 items=["TECH4.00", "TECH7.00", "TECH10.00", "NIST1.68", "NIST4.01", "NIST6.86", "NIST9.18", "NIST12.68"] ("标液2")
                w301 = u16 2 items=["TECH4.00", "TECH7.00", "TECH10.00", "NIST1.68", "NIST4.01", "NIST6.86", "NIST9.18", "NIST12.68"] ("标液3")
                w302 = u16 1 items=["TECH4.00", "TECH7.00", "TECH10.00", "NIST1.68", "NIST4.01", "NIST6.86", "NIST9.18", "NIST12.68"] ("标液2")
                n150 = local write "三点标液3"(w301) -> ()
                n151 = local write "三点标液2"(w302) -> ()
                n152 = local write "三点标液1"(w300) -> ()
              }
              frame 1 {
                w303 = u16 0 items=["TECH4.00", "TECH7.00", "TECH10.00", "NIST1.68", "NIST4.01", "NIST6.86", "NIST9.18", "NIST12.68"] ("标液2")
                w304 = u16 2 items=["TECH4.00", "TECH7.00", "TECH10.00", "NIST1.68", "NIST4.01", "NIST6.86", "NIST9.18", "NIST12.68"] ("标液3")
                w305 = u16 1 items=["TECH4.00", "TECH7.00", "TECH10.00", "NIST1.68", "NIST4.01", "NIST6.86", "NIST9.18", "NIST12.68"] ("标液2")
                n153 = local write "三点标液3"(w304) -> ()
                n154 = local write "三点标液2"(w305) -> ()
                n155 = local write "三点标液1"(w303) -> ()
              }
              frame 2 {
                w306 = u16 2 items=["TECH4.00", "TECH7.00", "TECH10.00", "NIST1.68", "NIST4.01", "NIST6.86", "NIST9.18", "NIST12.68"] ("标液2")
                w307 = u16 0 items=["TECH4.00", "TECH7.00", "TECH10.00", "NIST1.68", "NIST4.01", "NIST6.86", "NIST9.18", "NIST12.68"] ("标液3")
                w308 = u16 1 items=["TECH4.00", "TECH7.00", "TECH10.00", "NIST1.68", "NIST4.01", "NIST6.86", "NIST9.18", "NIST12.68"] ("标液2")
                n156 = local write "三点标液3"(w307) -> ()
                n157 = local write "三点标液2"(w308) -> ()
                n158 = local write "三点标液1"(w306) -> ()
              }
              frame 3 {
                w309 = u16 3 items=["TECH4.00", "TECH7.00", "TECH10.00", "NIST1.68", "NIST4.01", "NIST6.86", "NIST9.18", "NIST12.68"] ("标液2")
                w310 = u16 5 items=["TECH4.00", "TECH7.00", "TECH10.00", "NIST1.68", "NIST4.01", "NIST6.86", "NIST9.18", "NIST12.68"] ("标液3")
                w311 = u16 4 items=["TECH4.00", "TECH7.00", "TECH10.00", "NIST1.68", "NIST4.01", "NIST6.86", "NIST9.18", "NIST12.68"] ("标液2")
                n159 = local write "三点标液3"(w310) -> ()
                n160 = local write "三点标液2"(w311) -> ()
                n161 = local write "三点标液1"(w309) -> ()
              }
              frame 4 {
                w312 = u16 4 items=["TECH4.00", "TECH7.00", "TECH10.00", "NIST1.68", "NIST4.01", "NIST6.86", "NIST9.18", "NIST12.68"] ("标液2")
                w313 = u16 6 items=["TECH4.00", "TECH7.00", "TECH10.00", "NIST1.68", "NIST4.01", "NIST6.86", "NIST9.18", "NIST12.68"] ("标液3")
                w314 = u16 5 items=["TECH4.00", "TECH7.00", "TECH10.00", "NIST1.68", "NIST4.01", "NIST6.86", "NIST9.18", "NIST12.68"] ("标液2")
                n162 = local write "三点标液3"(w313) -> ()
                n163 = local write "三点标液2"(w314) -> ()
                n164 = local write "三点标液1"(w312) -> ()
              }
              frame 5..7 {
                w315 = u16 5 items=["TECH4.00", "TECH7.00", "TECH10.00", "NIST1.68", "NIST4.01", "NIST6.86", "NIST9.18", "NIST12.68"] ("标液2")
                w316 = u16 7 items=["TECH4.00", "TECH7.00", "TECH10.00", "NIST1.68", "NIST4.01", "NIST6.86", "NIST9.18", "NIST12.68"] ("标液3")
                w317 = u16 6 items=["TECH4.00", "TECH7.00", "TECH10.00", "NIST1.68", "NIST4.01", "NIST6.86", "NIST9.18", "NIST12.68"] ("标液2")
                n165 = local write "三点标液3"(w316) -> ()
                n166 = local write "三点标液2"(w317) -> ()
                n167 = local write "三点标液1"(w315) -> ()
              }
            }
            n168 = call "Add State to Queue.vi"("State(s) In (\"\")"=w296) -> ("States Out"=w297:string)  [unwired: 14 in]
          }
          event "三点标液2": Value Change {
            n169 = event-data() -> ("NewVal"=w321:u16)  [unwired: 1 in, 5 out]
            n170 = case shown="6, 7" w321 {
              frame 0..2, Default {
                w322 = u16 0 items=["TECH4.00", "TECH7.00", "TECH10.00", "NIST1.68", "NIST4.01", "NIST6.86", "NIST9.18", "NIST12.68"] ("标液2")
                w323 = u16 2 items=["TECH4.00", "TECH7.00", "TECH10.00", "NIST1.68", "NIST4.01", "NIST6.86", "NIST9.18", "NIST12.68"] ("标液3")
                w324 = u16 1 items=["TECH4.00", "TECH7.00", "TECH10.00", "NIST1.68", "NIST4.01", "NIST6.86", "NIST9.18", "NIST12.68"] ("标液2")
                n171 = local write "三点标液3"(w323) -> ()
                n172 = local write "三点标液2"(w324) -> ()
                n173 = local write "三点标液1"(w322) -> ()
              }
              frame 3, 4 {
                w325 = u16 3 items=["TECH4.00", "TECH7.00", "TECH10.00", "NIST1.68", "NIST4.01", "NIST6.86", "NIST9.18", "NIST12.68"] ("标液2")
                w326 = u16 5 items=["TECH4.00", "TECH7.00", "TECH10.00", "NIST1.68", "NIST4.01", "NIST6.86", "NIST9.18", "NIST12.68"] ("标液3")
                w327 = u16 4 items=["TECH4.00", "TECH7.00", "TECH10.00", "NIST1.68", "NIST4.01", "NIST6.86", "NIST9.18", "NIST12.68"] ("标液2")
                n174 = local write "三点标液3"(w326) -> ()
                n175 = local write "三点标液2"(w327) -> ()
                n176 = local write "三点标液1"(w325) -> ()
              }
              frame 5 {
                w328 = u16 6 items=["TECH4.00", "TECH7.00", "TECH10.00", "NIST1.68", "NIST4.01", "NIST6.86", "NIST9.18", "NIST12.68"] ("标液3")
                w329 = u16 5 items=["TECH4.00", "TECH7.00", "TECH10.00", "NIST1.68", "NIST4.01", "NIST6.86", "NIST9.18", "NIST12.68"] ("标液2")
                n177 = local write "三点标液3"(w328) -> ()
                n178 = local write "三点标液2"(w329) -> ()
              }
              frame 6, 7 {
                w330 = u16 7 items=["TECH4.00", "TECH7.00", "TECH10.00", "NIST1.68", "NIST4.01", "NIST6.86", "NIST9.18", "NIST12.68"] ("标液3")
                w331 = u16 6 items=["TECH4.00", "TECH7.00", "TECH10.00", "NIST1.68", "NIST4.01", "NIST6.86", "NIST9.18", "NIST12.68"] ("标液2")
                n179 = local write "三点标液3"(w330) -> ()
                n180 = local write "三点标液2"(w331) -> ()
              }
            }
            n181 = call "Add State to Queue.vi"("State(s) In (\"\")"=w318) -> ("States Out"=w319:string)  [unwired: 14 in]
          }
          event "三点标液3": Value Change {
            n182 = event-data() -> ("NewVal"=w335:u16)  [unwired: 1 in, 5 out]
            n183 = case shown="3..7" w335 {
              frame 0, 1, Default {
                w336 = u16 2 items=["TECH4.00", "TECH7.00", "TECH10.00", "NIST1.68", "NIST4.01", "NIST6.86", "NIST9.18", "NIST12.68"] ("标液2")
                w337 = u16 0 items=["TECH4.00", "TECH7.00", "TECH10.00", "NIST1.68", "NIST4.01", "NIST6.86", "NIST9.18", "NIST12.68"] ("标液3")
                w338 = u16 1 items=["TECH4.00", "TECH7.00", "TECH10.00", "NIST1.68", "NIST4.01", "NIST6.86", "NIST9.18", "NIST12.68"] ("标液2")
                n184 = local write "三点标液3"(w337) -> ()
                n185 = local write "三点标液2"(w338) -> ()
                n186 = local write "三点标液1"(w336) -> ()
              }
              frame 2 {
                w339 = u16 0 items=["TECH4.00", "TECH7.00", "TECH10.00", "NIST1.68", "NIST4.01", "NIST6.86", "NIST9.18", "NIST12.68"] ("标液2")
                w340 = u16 2 items=["TECH4.00", "TECH7.00", "TECH10.00", "NIST1.68", "NIST4.01", "NIST6.86", "NIST9.18", "NIST12.68"] ("标液3")
                w341 = u16 1 items=["TECH4.00", "TECH7.00", "TECH10.00", "NIST1.68", "NIST4.01", "NIST6.86", "NIST9.18", "NIST12.68"] ("标液2")
                n187 = local write "三点标液3"(w340) -> ()
                n188 = local write "三点标液2"(w341) -> ()
                n189 = local write "三点标液1"(w339) -> ()
              }
              frame 3..7 {
                n190 = local read "三点标液1"() -> (w344:u16)
                n191 = local read "三点标液2"() -> (w343:u16)
                n192 = Less?(x=w344, y=w343) -> (x < y?=w342:bool)
                n193 = case shown="假" w342 {
                  frame False {
                  }
                  frame True {
                    n194 = local read "三点标液3"() -> (w347:u16)
                    n195 = local read "三点标液2"() -> (w345:u16)
                    n196 = Less Or Equal?(x=w347, y=w345) -> (x <= y?=w346:bool)
                    n197 = case shown="真" w346 {
                      tunnel: w345 -> [_ w349]
                      frame False {
                      }
                      frame True {
                        n198 = Increment(x=w349) -> (x+1=w348:u16)
                        n199 = local write "三点标液3"(w348) -> ()
                      }
                    }
                  }
                }
              }
            }
            n200 = call "Add State to Queue.vi"("State(s) In (\"\")"=w332) -> ("States Out"=w333:string)  [unwired: 14 in]
          }
          event "标液1", "标液2", "偏移值补偿", "滤波设定": Mouse Down {
            n201 = event-data() -> ("CtlRef"=w356:refnum<vi>)  [unwired: 1 in, 7 out]
            n202 = property class="DigNum (严格)"(reference=w356) -> (reference out=w350:refnum<vi>, "Value"=w351:dbl)  [unwired: 1 in, 1 out]
            n203 = call "数字键盘.vi"("OldNumber"=w351) -> ("NewNumber"=w352:dbl)  [unwired: 1 in]
            n204 = property class="DigNum (严格)"(reference=w350, "Val(Sgnl)"=w352) -> ()  [unwired: 1 in, 2 out]
            n205 = call "Add State to Queue.vi"("State(s) In (\"\")"=w353) -> ("States Out"=w354:string)  [unwired: 14 in]
          }
          event "偏移值补偿": Value Change {
            n206 = event-data() -> ("NewVal"=w361:dbl)  [unwired: 1 in, 5 out]
            n207 = global read "多参数全局变量.vi" "MB session in"() -> (w362:refnum<class "MB_Master.lvclass">)
            n208 = call "000CH_pH_pH偏移修正值写入.vi"("数值"=w361, "MB session in"=w362) -> ("error out"=w359:errorcluster)  [unwired: 8 in, 1 out]
            n209 = Enqueue Element At Opposite End(queue=w360, element=通知队列类型."pH" ("枚举"), error in (no error)=w359) -> (error out=w358:errorcluster)  [unwired: 1 in, 2 out]
            n210 = call "Add State to Queue.vi"("State(s) In (\"\")"=w365) -> ("States Out"=w364:string)  [unwired: 14 in]
          }
          event "标液1": Value Change {
            n211 = event-data() -> ("NewVal"=w374:dbl)  [unwired: 1 in, 5 out]
            n212 = global read "多参数全局变量.vi" "MB session in"() -> (w372:refnum<class "MB_Master.lvclass">)
            n213 = call "0030H_pH_第一点标准值写入.vi"("数值"=w374, "MB session in"=w372) -> ("error out"=w373:errorcluster)  [unwired: 8 in, 1 out]
            n214 = Enqueue Element At Opposite End(queue=w367, element=通知队列类型."pH" ("枚举"), error in (no error)=w373) -> (error out=w368:errorcluster)  [unwired: 1 in, 2 out]
            n215 = call "Add State to Queue.vi"("State(s) In (\"\")"=w369) -> ("States Out"=w370:string)  [unwired: 14 in]
          }
          event "标液2": Value Change {
            n216 = event-data() -> ("NewVal"=w383:dbl)  [unwired: 1 in, 5 out]
            n217 = global read "多参数全局变量.vi" "MB session in"() -> (w381:refnum<class "MB_Master.lvclass">)
            n218 = call "0033H_pH_第二点标准值写入.vi"("数值"=w383, "MB session in"=w381) -> ("error out"=w382:errorcluster)  [unwired: 8 in, 1 out]
            n219 = Enqueue Element At Opposite End(queue=w376, element=通知队列类型."pH" ("枚举"), error in (no error)=w382) -> (error out=w377:errorcluster)  [unwired: 1 in, 2 out]
            n220 = call "Add State to Queue.vi"("State(s) In (\"\")"=w378) -> ("States Out"=w379:string)  [unwired: 14 in]
          }
          event "滤波设定": Value Change {
            n221 = event-data() -> ("NewVal"=w388:dbl)  [unwired: 1 in, 5 out]
            n222 = global read "多参数全局变量.vi" "MB session in"() -> (w389:refnum<class "MB_Master.lvclass">)
            n223 = call "0027H_pH_数位滤波设定写入.vi"("数值"=w388, "MB session in"=w389) -> ("error out"=w387:errorcluster)  [unwired: 8 in, 1 out]
            n224 = Enqueue Element At Opposite End(queue=w385, element=通知队列类型."pH" ("枚举"), error in (no error)=w387) -> (error out=w386:errorcluster)  [unwired: 1 in, 2 out]
            n225 = call "Add State to Queue.vi"("State(s) In (\"\")"=w390) -> ("States Out"=w391:string)  [unwired: 14 in]
          }
          event "刷新按钮": Value Change {
            n226 = event-data() -> ()  [unwired: 1 in, 6 out]
            n227 = call "Add State to Queue.vi"("State(s) In (\"\")"=w395) -> ("States Out"=w394:string)  [unwired: 14 in]
            n228 = Two Button Dialog(message="请再次确实是否恢复出厂设置！" ("消息")) -> (T button?=w397:bool)  [unwired: 2 in]
            n229 = case shown="真" w397 {
              frame False {
              }
              frame True {
                w398 = u16 33 items=["Factory Reset"=33] ("数值")
                n230 = global read "多参数全局变量.vi" "MB session in"() -> (w399:refnum<class "MB_Master.lvclass">)
                n231 = call "0026H_pH_命令寄存器写入.vi"("数值"=w398, "MB session in"=w399) -> ()  [unwired: 8 in, 2 out]
              }
            }
          }
          event "校准启动": Value Change {
            n232 = event-data() -> ()  [unwired: 1 in, 6 out]
            n233 = global read "多参数全局变量.vi" "校准运行状态"() -> (w401:T5)
            n234 = Bundle By Name(cluster=w401, "ph"=TRUE) -> (w402:T5)
            n235 = call "Add State to Queue.vi"("State(s) In (\"\")"=w406, "State(s) At Back (\"\")"="init: all\nCal: Place standard solution\n Cal: Calibration process\nidle" ("State(s) In (\"\")")) -> ("States Out"=w405:string)  [unwired: 13 in]
            n236 = global write "多参数全局变量.vi" "校准运行状态"(w402) -> ()
          }
          event "校准停止": Value Change {
            n237 = event-data() -> ()  [unwired: 1 in, 6 out]
            n238 = call "Add State to Queue.vi"("State(s) In (\"\")"="init: all\nCal: Over\nidle" ("State(s) In (\"\")")) -> ("States Out"=w408:string)  [unwired: 14 in]
          }
        }
      }
    }
  }
  n239 = while {
    stop <- FALSE stop-if-true
    n240 = global read "多参数全局变量.vi" "权限"() -> (w413:enum16{"一级权限", "二级权限", "三级权限"})
    n241 = Wait (ms)(milliseconds to wait=u32 1000 ("等待时间（毫秒）")) -> ()  [unwired: 1 out]
    n242 = Not Equal?(x=w413, y=enum16{"一级权限", "二级权限", "三级权限"}."一级权限") -> (x != y?=w410:bool)
    n243 = property on="滤波设定" class="DigNum (严格)"("Visible"=w410) -> ()  [unwired: 2 in, 2 out]
    n244 = property on="偏移值补偿" class="DigNum (严格)"("Visible"=w410) -> ()  [unwired: 2 in, 2 out]
  }
